vi "Split Panel.vi"(8 "error in (no error)":errorcluster caption="错误输入（无错误）", 10 "Split Mode":T1, 11 "PanelDataNode 输入":refnum<class "PanelDataNode.lvclass"> caption="DNL_LabVIEW Object in") -> (0 "error out":errorcluster caption="错误输出", 2 "ChildDataNode[]":refnum<data-value>[](array[refnum]), 3 "PanelDataNode 输出":refnum<class "PanelDataNode.lvclass"> caption="DNL_LabVIEW Object out")   [LabVIEW 2013, in "PanelDataNode.lvclass"]
uses:
  PanelDataNode.lvclass
  Split Mode.ctl
  PanelLinkNode/PanelLinkNode.lvclass/PanelLinkNode.ctl
  PanelObject/PanelObject.lvclass
  PanelLinkNode/PanelLinkNode.lvclass
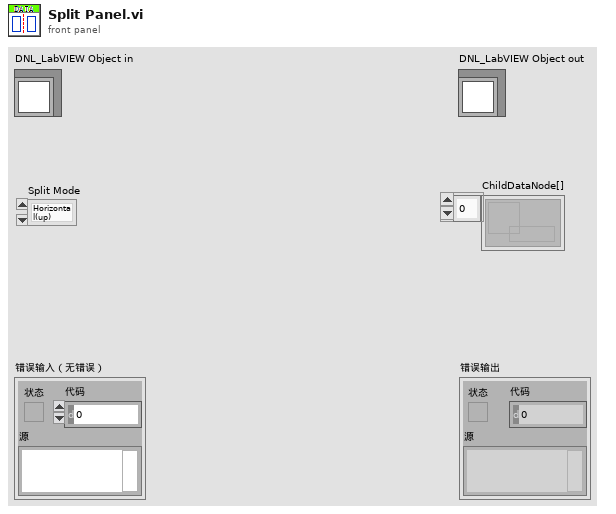
[diagram p1: front panel]
types:
  T1 = typedef "PanelDataNode.lvclass/Split Mode.ctl" = enum16{"Horizontal(up)", "Vertical(left)", "Horizontal(down)", "Vertical(right)"}
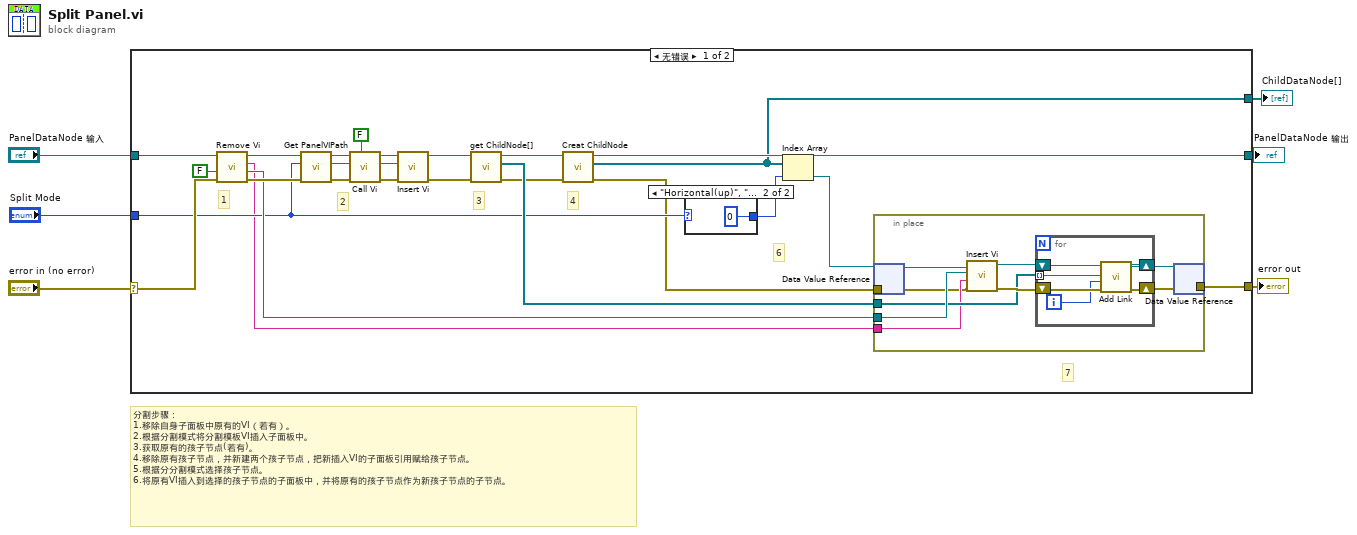
[diagram p0: block diagram]
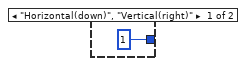
[diagram p2: hidden frame]
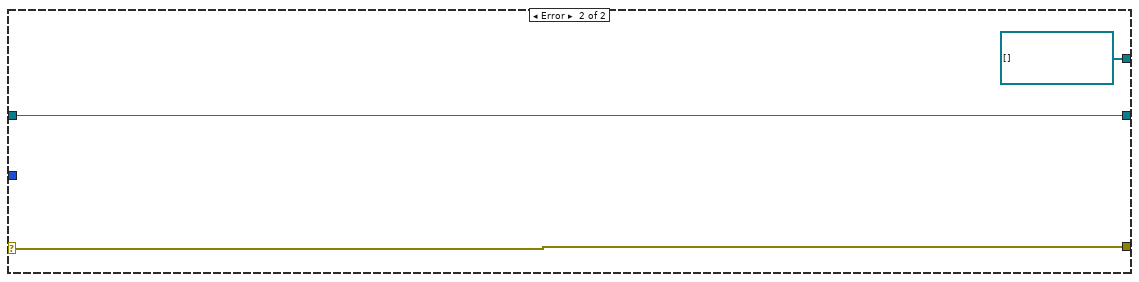
[diagram p3: hidden frame]
diagram:
  # "分割步骤：\n1.移除自身子面板中原有的VI（若有）。\n2.根据分割模式将分割模板VI插入子面板中。\n3.获取原有的孩子节点(若有)。\n4.移除原有孩子节点，并新建两个孩子节点，把新插入VI的子面板引用赋给孩子节点。\n5.根据分分割模式选择孩子节点。\n6.将原有VI插入到选择的孩子节点的子面板中，并将原有的孩子节点作为新孩子节点的子节点。"
  n1 = case shown="无错误" "error in (no error)" {
    selector: "error in (no error)" -> [w29 w52]
    tunnel: [w23 w52] -> w5
    tunnel: [w9 w51] -> w3
    tunnel: "PanelDataNode 输入" -> [w32 w51]
    tunnel: "Split Mode" -> [w19 _]
    tunnel: [w7 refnum<data-value>[] [] ("ChildDataNode[]")] -> w1
    frame No Error {
      # "7"
      # "6"
      # "4"
      # "3"
      # "2"
      # "1"
      n2 = call-dynamic "Remove Vi.vi"("error in"=w29, "Abort VI"=FALSE, "PanelDataNode 输入"=w32) -> ("error out"=w30:errorcluster, "VI*"=w27:refnum<vi>, "ViValue"=w8:string, "PanelDataNode 输出"=w31:refnum<class "PanelDataNode.lvclass">)  [unwired: 5 in]
      n3 = call-dynamic "Get PanelVIPath.vi"("error in (no error)"=w30, "Split Mode"=w19, "PanelDataNode 输入"=w31) -> ("error out"=w16:errorcluster, "panel path"=w13:path, "PanelDataNode 输出"=w18:refnum<class "PanelDataNode.lvclass">)  [unwired: 4 in]
      n4 = call-dynamic "Call Vi.vi"("Auto Dispose Ref"=FALSE, "error in (no error)"=w16, "Vi Path"=w13, "PanelDataNode 输入"=w18) -> ("error out"=w15:errorcluster, "VI*"=w14:refnum<vi>, "PanelDataNode 输出"=w17:refnum<class "PanelDataNode.lvclass">)  [unwired: 5 in]
      n5 = call-dynamic "Insert Vi.vi"("error in (no error)"=w15, "VI*"=w14, "PanelDataNode 输入"=w17) -> ("error out"=w25:errorcluster, "PanelDataNode 输出"=w26:refnum<class "PanelDataNode.lvclass">)  [unwired: 7 in]
      n6 = call "get ChildNode[].vi"("error in (no error)"=w25, "PanelLinkNode输入"=w26) -> ("error out"=w20:errorcluster, "ChildNode*[]"=w24:refnum<data-value>[], "PanelLinkNode输出"=w21:refnum<class "PanelDataNode.lvclass">)  [unwired: 7 in]
      n7 = call-dynamic "Creat ChildNode.vi"("error in"=w20, "ParentDataNode in"=w21) -> ("error out"=w12:errorcluster, "ChildDataNode[]"=w7:refnum<data-value>[], "ParentDataNode out"=w9:refnum<class "PanelDataNode.lvclass">)  [unwired: 7 in]
      n8 = case shown="\"Horizontal(up)\", \"Vertical(left)\", 默认" w19 {
        tunnel: [1 0] -> w10
        frame "Horizontal(down)", "Vertical(right)" {
        }
        frame "Horizontal(up)", "Vertical(left)", Default {
        }
      }
      n9 = Index Array(array=w7, index=w10) -> (element=w22:refnum<data-value>)
      n10 = in-place {
        in-place-border: w12 -> [w35]
        in-place-border: w27 -> [w43]
        in-place-border: w24 -> [w39]
        in-place-border: [w38] -> w23
        in-place-border: w8 -> [w37]
        n11 = in-place-dvr #1(w22) -> (w36:refnum<class "PanelDataNode.lvclass">)  [unwired: 1 out]
        n12 = call-dynamic "Insert Vi.vi"("error in (no error)"=w35, "ViValue"=w37, "VI*"=w43, "PanelDataNode 输入"=w36) -> ("error out"=w40:errorcluster, "PanelDataNode 输出"=w42:refnum<class "PanelDataNode.lvclass">)  [unwired: 6 in]
        n13 = for {
          shift-right: [w48] -> w41
          shift-left: w42 -> [w49]
          tunnel: w39 -> [w44] mode=indexing
          shift-right: [w46] -> w38
          shift-left: w40 -> [w47]
          i -> [w45]
          n14 = call-dynamic "Add Link.vi"("ParentLinkNode in"=w49, "ChildNode* in"=w44, "L\\R Child"=w45, "error in (no error)"=w47) -> ("ParentLinkNode out"=w48:refnum<class "PanelDataNode.lvclass">, "error out"=w46:errorcluster)  [unwired: 5 in]
        }
        n15 = in-place-dvr #1(w41) -> ()  [unwired: 2 out]
      }
    }
    frame Error {
    }
  }
  "error out" <- w5
  "PanelDataNode 输出" <- w3
  "ChildDataNode[]" <- w1
